vi "CheckIfStop.vi"(4 "AxisNumber":u8, 6 "NewPos-Data":T1, 8 "error in (no error)":errorcluster, 11 "CS++Motor in":refnum<class "CS++Motor.lvclass">) -> (0 "error out":errorcluster, 3 "CS++Motor out":refnum<class "CS++Motor.lvclass">)   [LabVIEW 2015, in "CS++Motor.lvlib" / "CS++Motor.lvclass"]
doc: "This VI sends the Movement Commands to the child class if necessary."
uses:
  CS++Motor.lvclass
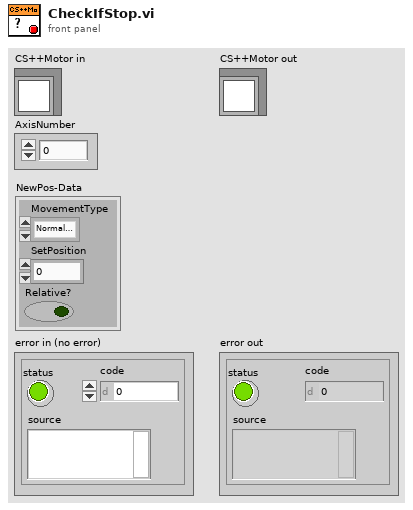
[diagram p1: front panel]
types:
  T1 = cluster{"MovementType":enum16{"NormalMovement", "ReferenceMovement", "StopMovement"}, "SetPosition":dbl, "Relative?":bool}
  T2 = enum16{"NormalMovement", "ReferenceMovement", "StopMovement"}
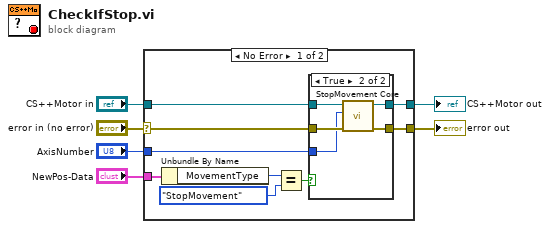
[diagram p0: block diagram]
diagram:
  n1 = case shown="No Error" "error in (no error)" {
    selector: "error in (no error)" -> [w12 w24]
    tunnel: [w10 w24] -> w5
    tunnel: [w11 w23] -> w1
    tunnel: "CS++Motor in" -> [w13 w23]
    tunnel: "AxisNumber" -> [w9 _]
    tunnel: "NewPos-Data" -> [w15 _]
    frame No Error {
      n2 = Unbundle By Name(w15) -> ("MovementType"=w14:T2)
      n3 = Equal?(x=w14, y=T2."StopMovement" ("MovementType")) -> (x = y?=w8:bool)
      n4 = case shown="True" w8 {
        tunnel: w13 -> [w17 w22]
        tunnel: w12 -> [w16 w21]
        tunnel: [w17 w20] -> w11
        tunnel: [w16 w19] -> w10
        tunnel: w9 -> [_ w18]
        frame False {
        }
        frame True {
          n5 = call-dynamic "StopMovement Core.vi"("error in (no error)"=w21, "AxisNumber"=w18, "CS++Motor in"=w22) -> ("error out"=w19:errorcluster, "CS++Motor out"=w20:refnum<class "CS++Motor.lvclass">)  [unwired: 7 in]
        }
      }
    }
    frame Error {
    }
  }
  "error out" <- w5
  "CS++Motor out" <- w1
